vi "Oxford-IPS120-Main.vi"() -> ()   [LabVIEW 2013]
uses:
  <instrlib>/Mercury iXX/Public/Libraries/System/Read/Time (Read).vi
  <instrlib>/Mercury iXX/Public/Libraries/Temperature/Open/Open Temperature Device.vi
  <instrlib>/Mercury iXX/Public/Libraries/Magnet/Open/Open Magnet Device.vi
  <instrlib>/Mercury iXX/Public/Libraries/Level Meter/Open/Open Level Meter Device.vi
  <instrlib>/Mercury iXX/Public/Libraries/Magnet/Signals/Read/Switch Heater Status (Read).vi
  <instrlib>/Mercury iXX/Public/Libraries/Magnet/Signals/Read/Current (Read).vi
  <instrlib>/Mercury iXX/Public/Libraries/Magnet/Signals/Read/Persistant Current (Read).vi
  <instrlib>/Mercury iXX/Public/Libraries/Magnet/Configuration/Set/PSU Action Status (Set).vi
  <instrlib>/Mercury iXX/Public/Libraries/Magnet/Controls/PSU Actions.ctl
  <instrlib>/Mercury iXX/Public/Libraries/Magnet/Controls/Switch Heater.ctl
  <instrlib>/Mercury iXX/Public/Libraries/Magnet/Signals/Set/Switch Heater No Check (Set).vi
  <instrlib>/Mercury iXX/Public/Libraries/Magnet/Signals/Set/Target Field Rate (Set).vi
  <instrlib>/Mercury iXX/Public/Libraries/Magnet/Signals/Set/Target Field (Set).vi
  <instrlib>/Mercury iXX/Private/Controls/Command Verbs.ctl
  <instrlib>/Mercury iXX/Public/Controls/ISOBus Address.ctl
  <userlib>/_OpenG.lib/error/error.llb/Filter Error Codes (Array)__ogtk.vi
  <instrlib>/Mercury iXX/Public/Controls/Unit String.ctl
  <instrlib>/Mercury iXX/Public/Libraries/System/Open/Open Device.vi
panel:
  in  "IPS120 Address":refnum<visa-resource-name>="GPIB1::25::INSTR"
  out "LPF ON":timestamp
  in  "Tab Control":T1(tab)
  in  "Set Needle Valve (%)":dbl format="%_2g"
  out "Sentinel":bool=TRUE
  in  "Remote Mode":bool
  out "Power Supply Field (T)":dbl=0.0001 format="%#.5f"
  out "Magnet Field (T)":dbl format="%.5f"
  out "Voltage (V)":dbl=-0.0003 format="%.5f"
  out "Current (A)":dbl=0.0006 format="%.5f"
  in  "Fast/Slow Fill":bool
  in  "OK":bool
  out "Magnet Field (T)":dbl(knob) caption="Voltage (V)" scale=-20.0..20.0
  out "Magnet Status 2":string
  out "Switch Time":string="11:11:48"
  in  "PS Heat":bool
  in  "Clamp":bool
  in  "To Set":bool
  in  "To Zero":bool
  in  "Hold":bool
  out "Magnet Status":string="Clamped"
  out "Target Field Rate (T/min)":dbl=1.0 format="%.5f"
  out "Target Field (T)":dbl format="%#.5f"
  in  "Target Rate (T/min)":dbl=0.1 format="%.5f"
  in  "Target Field (T)":dbl format="%#.5f"
  in  "Send to IPS":bool
  out "Voltage (V)":dbl(knob)=-0.0003 scale=-10.0..10.0
  out "Current (A)":dbl(knob)=0.0006 scale=-180.0..180.0
  out "Error List":T2(array[cluster])
  in  "Lambda":bool
  out "LPF on (s)":i32=5373
  # "Voltage (V)"
  # "Magnet (T)"
  # "Current (A)"
  # "Slow Rates\nCurrent Range (A)     Field Range (T)    Rate (T/min)\n0       -- 100        0    -- 11.5       0.91\n100     -- 150        11.5 -- 17.2       0.23\n150     -- 155.467    17.2 -- 18         0.11\n155.567 -- 172.471    18   -- 20         0.11\n\nFast Rates\nCurrent Range (A)     Field Range (T)    Rate (T/min)\n0       -- 155.467    0    -- 18         1.0\n155.567 -- 172.471    18   -- 20         0.25"
  # "This Control Doesn't Work"
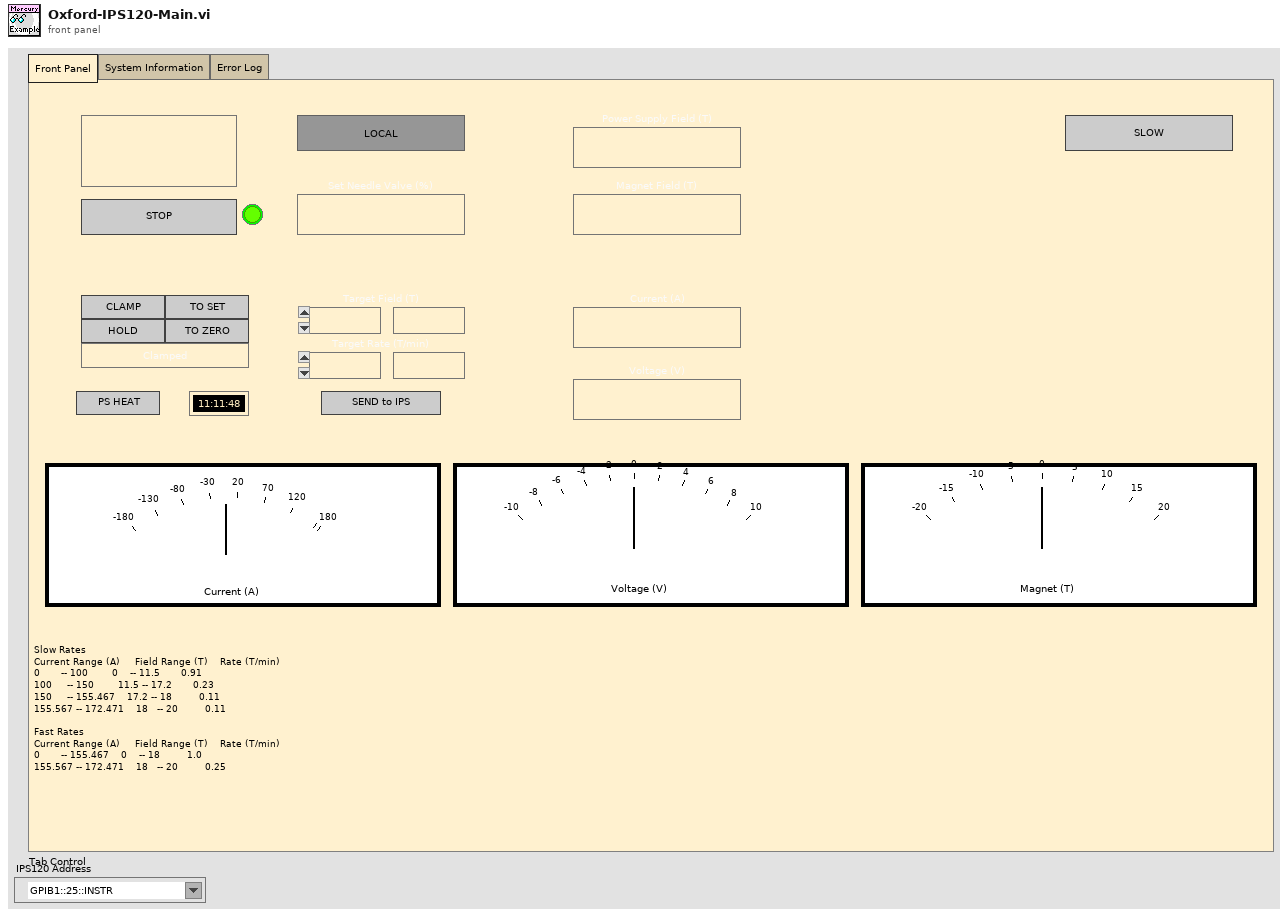
[diagram p1: front panel]
types:
  T1 = enum32{"Front Panel", "System Information", "Error Log"}
  T2 = cluster{"time":timestamp, "code":i32, "source":string}[]
  T3 = cluster{"Hold":bool, "Clamp":bool, "To Set":bool, "To Zero":bool, "Send to IPS":bool, "PS Heat":bool, "Lambda":bool}
  T4 = typedef "Mercury iXX.lvlib/Magnet.lvlib/PSU Actions.ctl" = string
  T5 = typedef "Mercury iXX.lvlib/Magnet.lvlib/Switch Heater.ctl" = string
  T6 = typedef "Mercury iXX.lvlib/Command Verbs.ctl" = string
  T7 = typedef "Mercury iXX.lvlib/ISOBus Address.ctl" = i32
  T8 = typedef "Mercury iXX.lvlib/Unit String.ctl" = string
  T9 = enum32{"invalid app kind", "Development System", "Run Time System", "Student Edition", "Embedded LabVIEW", "Evaluation", "Custom"}
  T10 = cluster{"time":timestamp, "code":i32, "source":string}
  T11 = enum32{"Invalid", "Standard", "Closed", "Hidden", "Minimized", "Maximized"}
  T12 = cluster{"Core":cluster{"Current VI Reference":refnum<vi>, "Close Panel on Exit?":bool}, "IPS120 Address":refnum<visa-resource-name>, "sentinel":bool, "Error Log":cluster{"time":timestamp, "code":i32, "source":string}[]}
  T13 = typedef "Mercury iXX.lvlib/Mercury Reference.ctl" = cluster{"Comms":refnum<visa-resource-name>, "Device ID":string[], "Comms Layer":T14, "Command":string, "Query reference":T15}
  T14 = typedef "Mercury iXX.lvlib/Comms Transport Layer.ctl" = enum16{"Ethernet TCP/IP", "USB", "ISOBus - RS-232", "GPIB"}
  T15 = typedef "Mercury iXX.lvlib/Query Dynamic Reference.ctl" = refnum<vi>
  T16 = typedef "Mercury iXX.lvlib/Response String.ctl" = string
  T17 = cluster{"Target Field (T)":dbl, "Target Field Rate (T/min)":dbl}
  T18 = typedef "Filtered Error Details - Cluster__ogtk.ctl" = cluster{"code":i32, "source":string}
  T19 = cluster{"Current VI Reference":refnum<vi>, "Close Panel on Exit?":bool}
  T20 = cluster{"Magnet Field":dbl, "PS Field":dbl, "Target Field":dbl, "Target Field Rate":dbl, "Voltage":dbl, "Current":dbl, "Switch":bool}
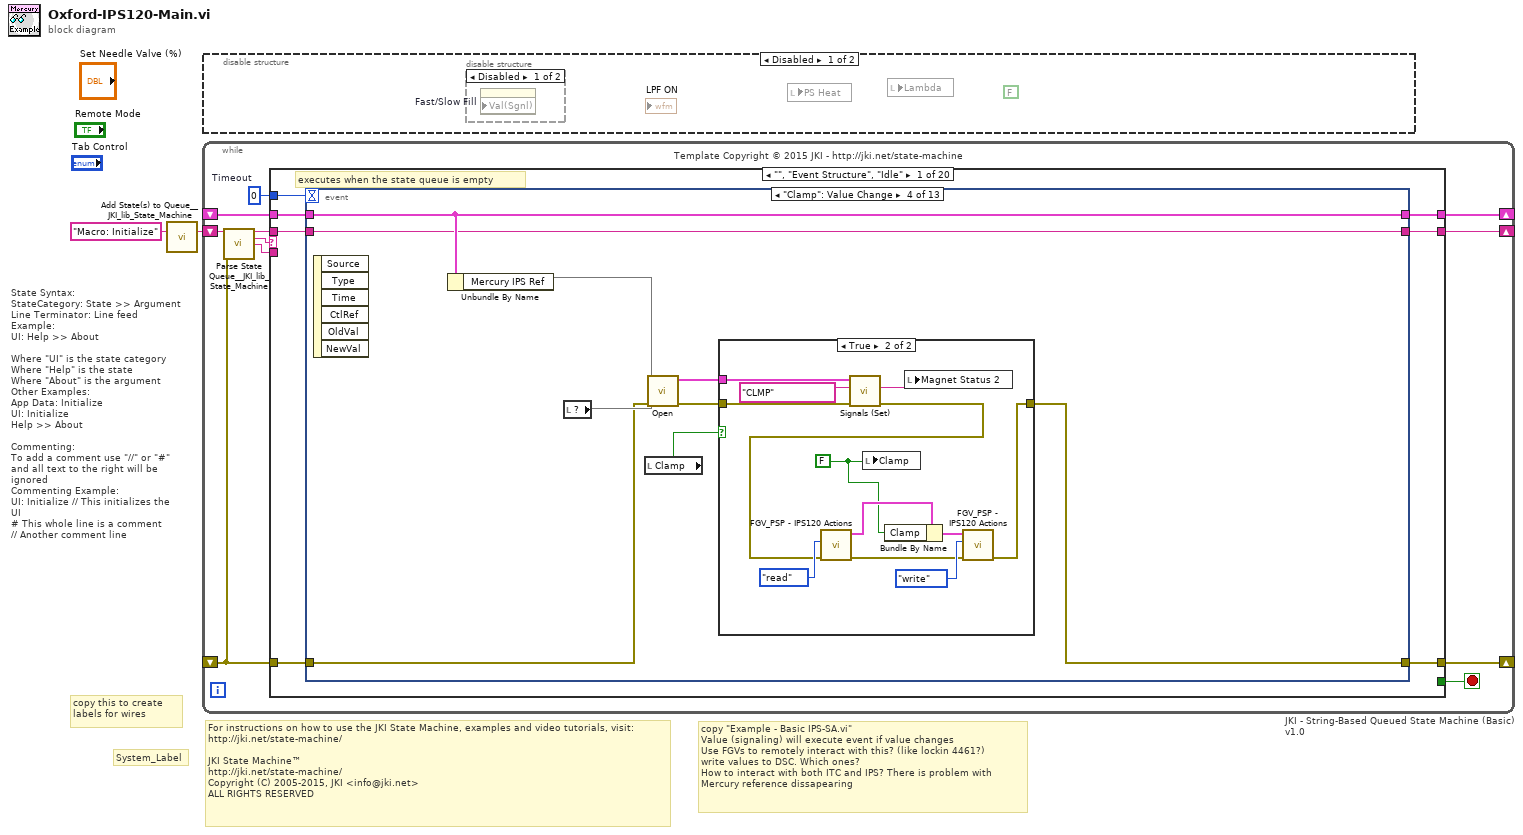
[diagram p0: block diagram]
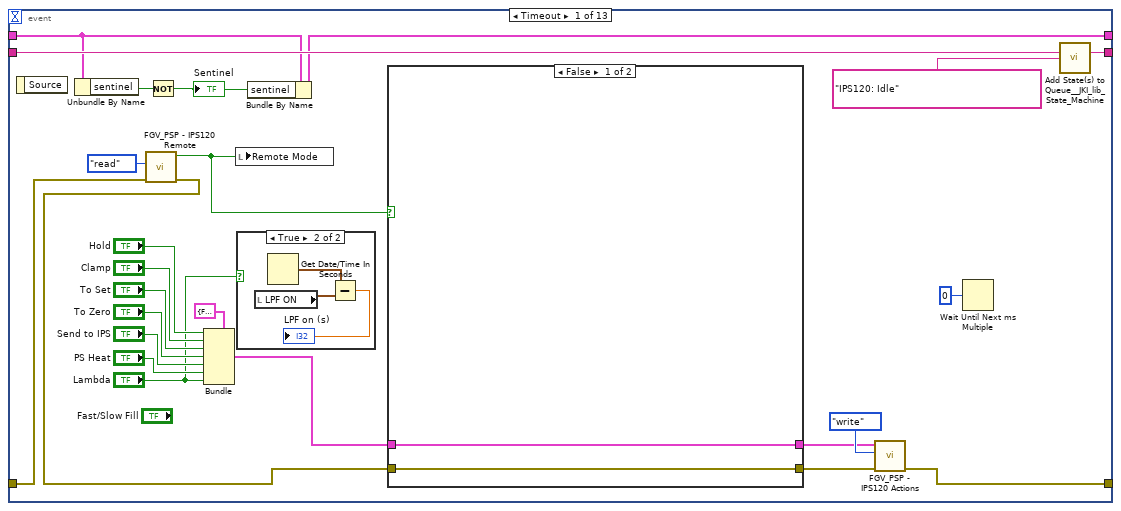
[diagram p4: hidden frame]
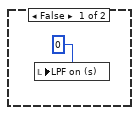
[diagram p5: hidden frame]
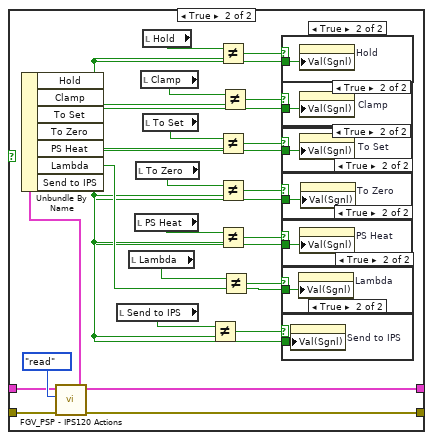
[diagram p6: hidden frame]
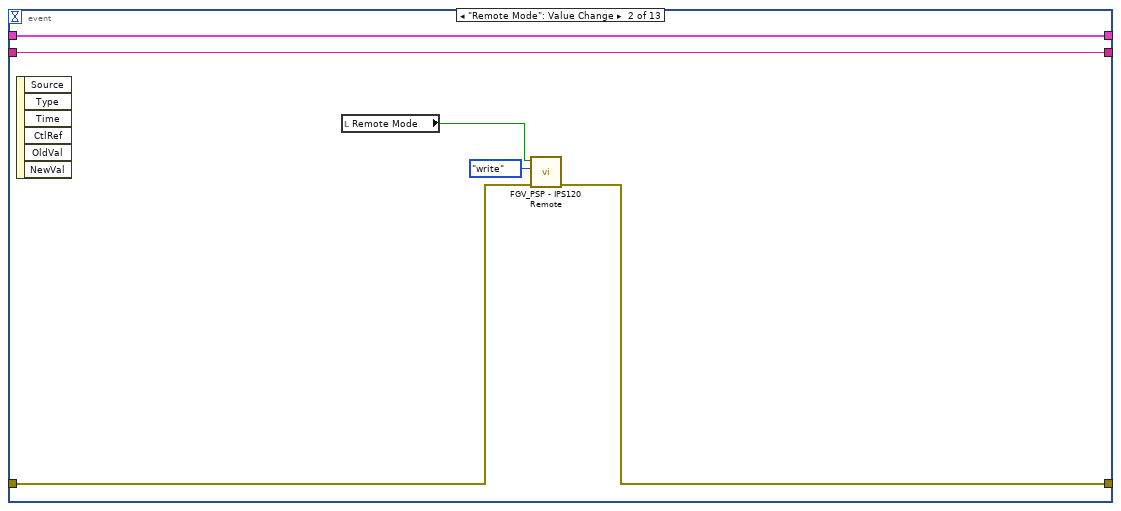
[diagram p14: hidden frame]
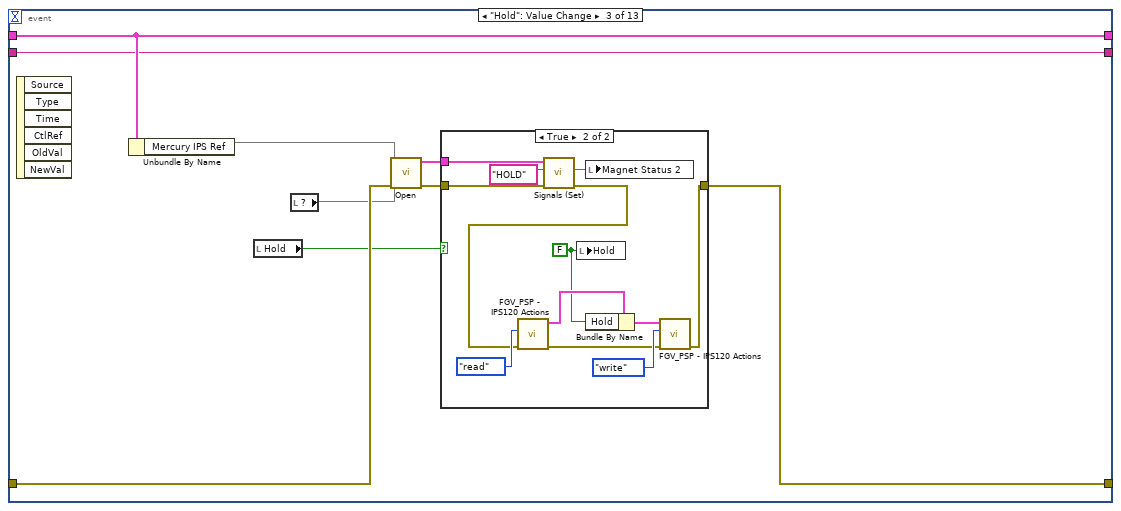
[diagram p15: hidden frame]
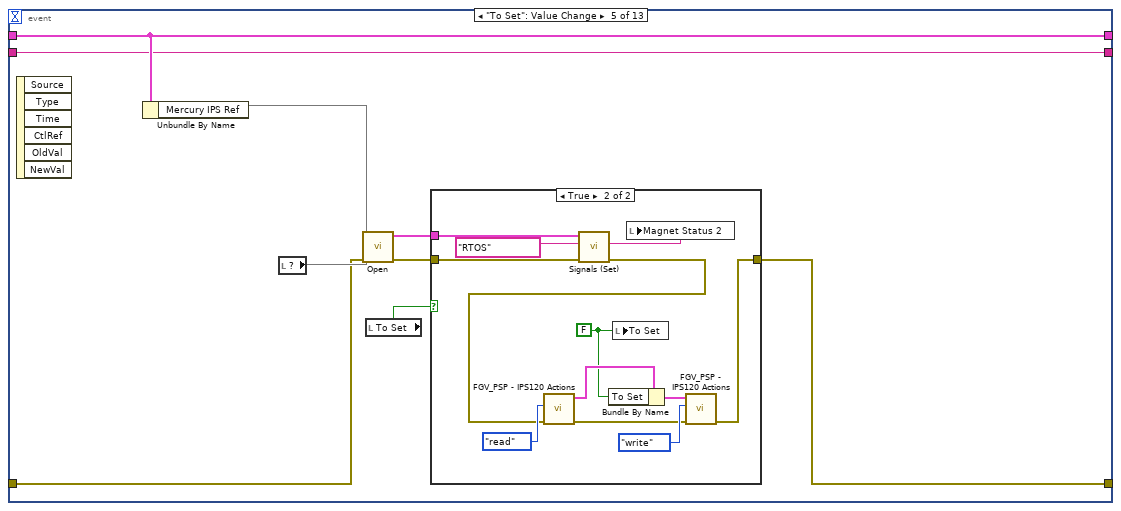
[diagram p18: hidden frame]
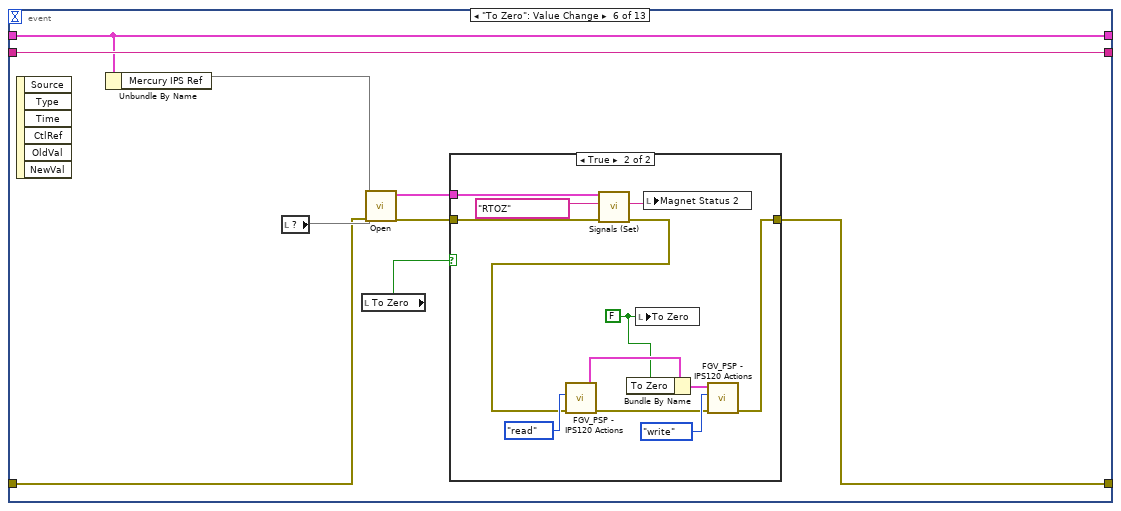
[diagram p20: hidden frame]
diagram:
  # "copy \"Example - Basic IPS-SA.vi\"\nValue (signaling) will execute event if value changes\nUse FGVs to remotely interact with this? (like lockin 4461?)\nwrite values to DSC. Which ones?\nHow to interact with both ITC and IPS? There is problem with \nMercury reference dissapearing"
  # "For instructions on how to use the JKI State Machine, examples and video tutorials, visit:\nhttp://jki.net/state-machine/\n\nJKI State Machine™\nhttp://jki.net/state-machine/\nCopyright (C) 2005-2015, JKI <info@jki.net>\nALL RIGHTS RESERVED"
  # "State Syntax:\nStateCategory: State >> Argument\nLine Terminator: Line feed\nExample:\nUI: Help >> About\n\nWhere \"UI\" is the state category\nWhere \"Help\" is the state\nWhere \"About\" is the argument\nOther Examples:\nApp Data: Initialize\nUI: Initialize\nHelp >> About\n\nCommenting:\nTo add a comment use \"//\" or \"#\" and all text to the right will be ignored\nCommenting Example:\nUI: Initialize // This initializes the UI\n# This whole line is a comment\n// Another comment line"
  # "copy this to create labels for wires"
  # "System_Label"
  n1 = call <vilib>:"Add State(s) to Queue__JKI_lib_State_Machine.vi"("State(s) in (\"\")"="Macro: Initialize") -> ("States Out"=w2:string)  [unwired: 14 in]
  n2 = while "JKI - String-Based Queued State Machine (Basic) v1.0" {
    shift-right: [w6] -> _
    shift-left: _ -> [w5]
    shift-right: [w9] -> _
    shift-left: _ -> [w3]
    shift-right: [w8] -> _
    shift-left: w2 -> [w10]
    stop <- w7 stop-if-true
    w4 = 0  # Timeout
    # "Template Copyright © 2015 JKI - http://jki.net/state-machine"
    n3 = call <vilib>:"Parse State Queue__JKI_lib_State_Machine.vi"("State Queue"=w10, "Error In (no error)"=w3) -> ("Remaining States"=w12:string, "Current State"=w13:string, "Arguments"=w11:string)  [unwired: 11 in]
    n4 = case shown="\"\", \"Event Structure\", \"Idle\"" w13 {
      selector: w13 -> [_ _ w361 _ _ _ _ _ _ _ _ _ _ _ _ _ _ _ _ _]
      tunnel: w12 -> [w20 w360 w365 w383 w400 w405 w409 w417 w423 w427 w439 w446 w457 w483 w488 w503 w507 w516 w551 w555]
      tunnel: w11 -> [_ _ _ _ _ _ _ _ _ _ _ w441 w451 _ _ _ _ _ _ _]
      tunnel: w5 -> [w16 w357 w363 w374 w386 w403 w406 _ w418 w424 w437 w444 w453 w480 w486 w501 w504 w514 w550 w554]
      tunnel: [w14 w358 w367 w380 errorcluster {"status"=FALSE, "code"=0, "source"=""} ("error out") w402 w407 w412 w419 w425 w433 w442 w454 w481 w485 w489 w505 w510 w546 w553] -> w9
      tunnel: [w19 w359 w364 w382 w399 w404 w408 w416 w422 w426 w438 w445 w456 w482 w487 w502 w506 w515 w552 w556] -> w8
      tunnel: [_ _ _ _ _ TRUE _ _ _ _ _ _ _ _ _ _ _ _ _ _] -> w7
      tunnel: [w18 w357 w363 w381 w385 w403 w406 w415 w418 w424 w437 w444 w453 w480 w486 w501 w504 w513 w550 w554] -> w6
      tunnel: w4 -> [w17 _ _ _ _ _ _ _ _ _ _ _ _ _ _ _ _ _ _ _]
      tunnel: w3 -> [w15 w358 w366 w380 w395 w402 w407 w412 w420 w425 w429 w443 w455 w481 w485 w491 w505 w511 w523 w553]
      frame "", "Event Structure", "Idle" {
        # "executes when the state queue is empty"
        n5 = event shown="[3] \"Clamp\": Value Change" {
          selector: _ -> [_ _ _ _ _ _ _ _ _ _ _ _ _]
          dyn-events: _ -> [_ _ _ _ _ _ _ _ _ _ _ _ _]
          timeout: w17 -> [_ _ _ _ _ _ _ _ _ _ _ _ _]
          tunnel: w20 -> [w45 w87 w98 w120 w141 w164 w190 w254 w285 w326 w329 w350 w356]
          tunnel: [w44 w87 w98 w120 w141 w164 w190 w254 w285 w326 w329 w349 w355] -> w19
          tunnel: [w39 w86 w99 w121 w142 w163 w191 w250 w284 w318 w344 w347 w353] -> w18
          tunnel: w16 -> [w40 w86 w99 w121 w142 w163 w191 w250 w284 w318 w344 w347 w353]
          tunnel: w15 -> [w23 w89 w95 w116 w136 w158 w184 w253 w282 w323 w331 w348 w354]
          tunnel: [w33 w88 w97 w113 w143 w165 w189 w251 w281 w306 w332 w348 w354] -> w14
          event Timeout {
            n6 = event-data() -> ()  [unwired: 1 in, 1 out]
            n7 = Unbundle By Name(w40) -> ("sentinel"=w42:bool)
            n8 = call "FGV_PSP - IPS120 Remote.vi"("error in"=w23, "Function"=enum16{"write", "read"}."read") -> ("error out"=w22:errorcluster, "Mercury Remote"=w21:bool)  [unwired: 4 in]
            n9 = Not(x=w42) -> (.not. x?=w41:bool)
            "Sentinel" <- w41
            n10 = Bundle(cluster=T3 {"Hold"=FALSE, "Clamp"=FALSE, "To Set"=FALSE, "To Zero"=FALSE, "Send to IPS"=FALSE, "PS Heat"=FALSE, "Lambda"=FALSE}, "Hold"="Hold", "Clamp"="Clamp", "To Set"="To Set", "To Zero"="To Zero", "Send to IPS"="Send to IPS", "PS Heat"="PS Heat", "Lambda"="Lambda") -> (w31:T3)
            n11 = local write "Remote Mode"(w21) -> ()
            n12 = case shown="True" "Lambda" {
              frame False {
                n13 = local write "LPF on (s)"(0 ("LPF on (s)")) -> ()
              }
              frame True {
                n14 = local read "LPF ON"() -> (w49:timestamp)
                n15 = Get Date/Time In Seconds() -> (seconds since 1Jan1904=w48:timestamp)
                n16 = Subtract(x=w48, y=w49) -> (x-y=→"LPF on (s)":dbl)
              }
            }
            n17 = Bundle By Name(cluster=w40, "sentinel"=w41) -> (w39:T12)
            n18 = case shown="False" w21 {
              tunnel: [w50 w76] -> w32
              tunnel: w22 -> [w50 w75]
              tunnel: w31 -> [w51 w74]
              tunnel: [w51 w66] -> w30
              frame False {
              }
              frame True {
                n19 = call "FGV_PSP - IPS120 Actions.vi"("error in"=w75, "Function"=enum16{"write", "read"}."read", "mercury actions"=w74) -> ("error out"=w76:errorcluster, "mercury actions 2"=w66:T3)  [unwired: 3 in]
                n20 = Unbundle By Name(w66) -> ("Hold"=w58:bool, "Clamp"=w60:bool, "To Set"=w61:bool, "To Zero"=w62:bool, "PS Heat"=w63:bool, "Lambda"=w64:bool, "Send to IPS"=w65:bool)
                n21 = local read "Send to IPS"() -> (w59:bool)
                n22 = local read "Lambda"() -> (w57:bool)
                n23 = local read "PS Heat"() -> (w56:bool)
                n24 = local read "To Zero"() -> (w55:bool)
                n25 = local read "Clamp"() -> (w53:bool)
                n26 = local read "Hold"() -> (w52:bool)
                n27 = local read "To Set"() -> (w54:bool)
                n28 = Not Equal?(x=w59, y=w65) -> (x != y?=w67:bool)
                n29 = Not Equal?(x=w52, y=w58) -> (x != y?=w73:bool)
                n30 = Not Equal?(x=w54, y=w61) -> (x != y?=w71:bool)
                n31 = Not Equal?(x=w55, y=w62) -> (x != y?=w70:bool)
                n32 = Not Equal?(x=w56, y=w63) -> (x != y?=w69:bool)
                n33 = Not Equal?(x=w53, y=w60) -> (x != y?=w72:bool)
                n34 = Not Equal?(x=w57, y=w64) -> (x != y?=w68:bool)
                n35 = case shown="True" w73 {
                  tunnel: w58 -> [_ w84]
                  frame False {
                  }
                  frame True {
                    n36 = property on="Hold" class="Bool (strict)"("Val(Sgnl)"=w84) -> ()  [unwired: 2 in, 2 out]
                  }
                }
                n37 = case shown="True" w72 {
                  tunnel: w60 -> [_ w83]
                  frame False {
                  }
                  frame True {
                    n38 = property on="Clamp" class="Bool (strict)"("Val(Sgnl)"=w83) -> ()  [unwired: 2 in, 2 out]
                  }
                }
                n39 = case shown="True" w71 {
                  tunnel: w61 -> [_ w82]
                  frame False {
                  }
                  frame True {
                    n40 = property on="To Set" class="Bool (strict)"("Val(Sgnl)"=w82) -> ()  [unwired: 2 in, 2 out]
                  }
                }
                n41 = case shown="True" w70 {
                  tunnel: w62 -> [_ w81]
                  frame False {
                  }
                  frame True {
                    n42 = property on="To Zero" class="Bool (strict)"("Val(Sgnl)"=w81) -> ()  [unwired: 2 in, 2 out]
                  }
                }
                n43 = case shown="True" w69 {
                  tunnel: w63 -> [_ w80]
                  frame False {
                  }
                  frame True {
                    n44 = property on="PS Heat" class="Bool (strict)"("Val(Sgnl)"=w80) -> ()  [unwired: 2 in, 2 out]
                  }
                }
                n45 = case shown="True" w68 {
                  tunnel: w64 -> [_ w79]
                  frame False {
                  }
                  frame True {
                    n46 = property on="Lambda" class="Bool (strict)"("Val(Sgnl)"=w79) -> ()  [unwired: 2 in, 2 out]
                  }
                }
                n47 = case shown="True" w67 {
                  tunnel: w65 -> [_ w78]
                  frame False {
                  }
                  frame True {
                    n48 = property on="Send to IPS" class="Bool (strict)"("Val(Sgnl)"=w78) -> ()  [unwired: 2 in, 2 out]
                  }
                }
              }
            }
            n49 = call "FGV_PSP - IPS120 Actions.vi"("error in"=w32, "Function"=enum16{"write", "read"}."write", "mercury actions"=w30) -> ("error out"=w33:errorcluster)  [unwired: 3 in, 1 out]
            n50 = Wait Until Next ms Multiple(millisecond multiple=u32 0) -> ()  [unwired: 1 out]
            n51 = call <vilib>:"Add State(s) to Queue__JKI_lib_State_Machine.vi"("State(s) in (\"\")"=w45, "State(s) at Back (\"\")"="IPS120: Idle" ("State(s) at Back (\"\")")) -> ("States Out"=w44:string)  [unwired: 13 in]
          }
          event "Remote Mode": Value Change {
            n52 = event-data() -> ()  [unwired: 1 in, 6 out]
            n53 = local read "Remote Mode"() -> (w85:bool)
            n54 = call "FGV_PSP - IPS120 Remote.vi"("error in"=w89, "Function"=enum16{"write", "read"}."write", "Mercury Remote"=w85) -> ("error out"=w88:errorcluster)  [unwired: 3 in, 1 out]
          }
          event "Hold": Value Change {
            n55 = event-data() -> ()  [unwired: 1 in, 6 out]
            n56 = Unbundle By Name(w99) -> ("Mercury IPS Ref"=w93)
            n57 = local read "Hold"() -> (w91:bool)
            n58 = local read item#-1() -> (w94)
            n59 = call-poly <instrlib>:"Open.vi"("error in (no error)"=w95, "Device Identifier"=w94, "Mercury Reference In"=w93) -> ("error out"=w96:errorcluster, "Mercury Reference Out"=w92:T13)  [unwired: 7 out]
            n60 = case shown="True" w91 {
              tunnel: [w100 w102] -> w97
              tunnel: w96 -> [w100 w111]
              tunnel: w92 -> [_ w110]
              frame False {
              }
              frame True {
                w107 = FALSE ("Hold")
                n61 = call-poly <instrlib>:"Signals (Set).vi"("error in"=w111, "PSU Act Stat"=T4 "HOLD", "Mercury Reference In"=w110) -> ("error out"=w101:errorcluster, "Response"=w109:T16)  [unwired: 1 in, 6 out]
                n62 = call "FGV_PSP - IPS120 Actions.vi"("error in"=w101, "Function"=enum16{"write", "read"}."read") -> ("error out"=w104:errorcluster, "mercury actions 2"=w108:T3)  [unwired: 4 in]
                n63 = local write "Hold"(w107) -> ()
                n64 = local write "Magnet Status 2"(w109) -> ()
                n65 = Bundle By Name(cluster=w108, "Hold"=w107) -> (w106:T3)
                n66 = call "FGV_PSP - IPS120 Actions.vi"("error in"=w104, "Function"=enum16{"write", "read"}."write", "mercury actions"=w106) -> ("error out"=w102:errorcluster)  [unwired: 3 in, 1 out]
              }
            }
          }
          event "Clamp": Value Change {
            n67 = event-data() -> ()  [unwired: 1 in, 6 out]
            n68 = Unbundle By Name(w121) -> ("Mercury IPS Ref"=w115)
            n69 = local read item#-1() -> (w119)
            n70 = local read "Clamp"() -> (w114:bool)
            n71 = call-poly <instrlib>:"Open.vi"("error in (no error)"=w116, "Device Identifier"=w119, "Mercury Reference In"=w115) -> ("error out"=w118:errorcluster, "Mercury Reference Out"=w117:T13)  [unwired: 7 out]
            n72 = case shown="True" w114 {
              tunnel: w118 -> [w122 w132]
              tunnel: w117 -> [_ w131]
              tunnel: [w122 w124] -> w113
              frame False {
              }
              frame True {
                w123 = FALSE
                n73 = call-poly <instrlib>:"Signals (Set).vi"("error in"=w132, "PSU Act Stat"=T4 "CLMP", "Mercury Reference In"=w131) -> ("error out"=w125:errorcluster, "Response"=w133:T16)  [unwired: 1 in, 6 out]
                n74 = call "FGV_PSP - IPS120 Actions.vi"("error in"=w125, "Function"=enum16{"write", "read"}."read") -> ("error out"=w127:errorcluster, "mercury actions 2"=w130:T3)  [unwired: 4 in]
                n75 = local write "Clamp"(w123) -> ()
                n76 = Bundle By Name(cluster=w130, "Clamp"=w123) -> (w129:T3)
                n77 = local write "Magnet Status 2"(w133) -> ()
                n78 = call "FGV_PSP - IPS120 Actions.vi"("error in"=w127, "Function"=enum16{"write", "read"}."write", "mercury actions"=w129) -> ("error out"=w124:errorcluster)  [unwired: 3 in, 1 out]
              }
            }
          }
          event "To Set": Value Change {
            n79 = event-data() -> ()  [unwired: 1 in, 6 out]
            n80 = Unbundle By Name(w142) -> ("Mercury IPS Ref"=w138)
            n81 = local read item#-1() -> (w137)
            n82 = call-poly <instrlib>:"Open.vi"("error in (no error)"=w136, "Device Identifier"=w137, "Mercury Reference In"=w138) -> ("error out"=w139:errorcluster, "Mercury Reference Out"=w140:T13)  [unwired: 7 out]
            n83 = local read "To Set"() -> (w135:bool)
            n84 = case shown="True" w135 {
              tunnel: [w144 w146] -> w143
              tunnel: w140 -> [_ w154]
              tunnel: w139 -> [w144 w153]
              frame False {
              }
              frame True {
                w145 = FALSE
                n85 = call-poly <instrlib>:"Signals (Set).vi"("error in"=w153, "PSU Act Stat"=T4 "RTOS", "Mercury Reference In"=w154) -> ("error out"=w147:errorcluster, "Response"=w155:T16)  [unwired: 1 in, 6 out]
                n86 = call "FGV_PSP - IPS120 Actions.vi"("error in"=w147, "Function"=enum16{"write", "read"}."read") -> ("error out"=w149:errorcluster, "mercury actions 2"=w152:T3)  [unwired: 4 in]
                n87 = Bundle By Name(cluster=w152, "To Set"=w145) -> (w151:T3)
                n88 = local write "To Set"(w145) -> ()
                n89 = local write "Magnet Status 2"(w155) -> ()
                n90 = call "FGV_PSP - IPS120 Actions.vi"("error in"=w149, "Function"=enum16{"write", "read"}."write", "mercury actions"=w151) -> ("error out"=w146:errorcluster)  [unwired: 3 in, 1 out]
              }
            }
          }
          event "To Zero": Value Change {
            n91 = event-data() -> ()  [unwired: 1 in, 6 out]
            n92 = Unbundle By Name(w163) -> ("Mercury IPS Ref"=w160)
            n93 = local read item#-1() -> (w159)
            n94 = local read "To Zero"() -> (w157:bool)
            n95 = call-poly <instrlib>:"Open.vi"("error in (no error)"=w158, "Device Identifier"=w159, "Mercury Reference In"=w160) -> ("error out"=w161:errorcluster, "Mercury Reference Out"=w162:T13)  [unwired: 7 out]
            n96 = case shown="True" w157 {
              tunnel: [w166 w169] -> w165
              tunnel: w162 -> [_ w176]
              tunnel: w161 -> [w166 w175]
              frame False {
              }
              frame True {
                w167 = FALSE
                n97 = call-poly <instrlib>:"Signals (Set).vi"("error in"=w175, "PSU Act Stat"=T4 "RTOZ", "Mercury Reference In"=w176) -> ("error out"=w170:errorcluster, "Response"=w177:T16)  [unwired: 1 in, 6 out]
                n98 = call "FGV_PSP - IPS120 Actions.vi"("error in"=w170, "Function"=enum16{"write", "read"}."read") -> ("error out"=w172:errorcluster, "mercury actions 2"=w168:T3)  [unwired: 4 in]
                n99 = Bundle By Name(cluster=w168, "To Zero"=w167) -> (w174:T3)
                n100 = local write "To Zero"(w167) -> ()
                n101 = local write "Magnet Status 2"(w177) -> ()
                n102 = call "FGV_PSP - IPS120 Actions.vi"("error in"=w172, "Function"=enum16{"write", "read"}."write", "mercury actions"=w174) -> ("error out"=w169:errorcluster)  [unwired: 3 in, 1 out]
              }
            }
          }
          event "PS Heat": Value Change {
            n103 = event-data() -> ()  [unwired: 1 in, 6 out]
            n104 = local read item#-1() -> (w185)
            n105 = Unbundle By Name(w191) -> ("Mercury IPS Ref"=w187)
            n106 = call-poly <instrlib>:"Open.vi"("error in (no error)"=w184, "Device Identifier"=w185, "Mercury Reference In"=w187) -> ("error out"=w181:errorcluster, "Mercury Reference Out"=w182:T13)  [unwired: 7 out]
            n107 = call-poly <instrlib>:"Signals (Read).vi"("error in"=w181, "Mercury Reference In"=w182) -> ("error out"=w193:errorcluster, "Current"=w188:dbl, "Mercury Reference Out"=w192:T13)  [unwired: 1 in, 6 out]
            n108 = local read "PS Heat"() -> (w180:bool)
            n109 = call-poly <instrlib>:"Signals (Read).vi"("error in"=w193, "Mercury Reference In"=w192) -> ("error out"=w194:errorcluster, "Persistant Current"=w183:dbl, "Mercury Reference Out"=w195:T13)  [unwired: 1 in, 6 out]
            n110 = Subtract(x=w183, y=w188) -> (x-y=w196:dbl)
            n111 = Absolute Value(x=w196) -> (abs(x)=w197:dbl)
            n112 = Less?(x=w197, y=0.1) -> (x < y?=w199:bool)
            n113 = case shown="False" w199 {
              selector: w199 -> [_ w202]
              tunnel: [w201 w202] -> w179
              frame False {
                n114 = Two Button Dialog(message="The magnet current is more\nthan 0.1A different to the\nPSU output current.  It is not\nadvisable to switch on the\nswitch heater unless these\ncurrents are equal!") -> (T button?=w201:bool)  [unwired: 2 out]
              }
              frame True {
              }
            }
            n115 = And(x=w180, y=w179) -> (x .and. y?=w186:bool)
            n116 = case shown="True" w186 {
              tunnel: w195 -> [_ w213]
              tunnel: w194 -> [w203 w212]
              tunnel: [w203 w204] -> w189
              frame False {
              }
              frame True {
                w206 = FALSE
                n117 = flat-sequence {
                  tunnel: [w224] -> w221
                  tunnel: [w223] -> w220
                  tunnel: [w222] -> w219
                  tunnel: w213 -> [w226]
                  tunnel: w212 -> [w225]
                  tunnel: w221 -> [w229]
                  tunnel: w220 -> [w228]
                  tunnel: [w229] -> w218
                  tunnel: [w228] -> w217
                  tunnel: [w227] -> w216
                  tunnel: w219 -> [w227]
                  tunnel: w218 -> [w240]
                  tunnel: w217 -> [w241]
                  tunnel: w216 -> [w238]
                  tunnel: [w235] -> w215
                  tunnel: [w236] -> w214
                  tunnel: w215 -> [w245]
                  tunnel: w214 -> [w244]
                  tunnel: [w243] -> w205
                  frame #0 {
                    n118 = call-poly <instrlib>:"Signals (Read).vi"("error in"=w225, "Mercury Reference In"=w226) -> ("error out"=w224:errorcluster, "Switch Heater Status"=w222:string, "Mercury Reference Out"=w223:T13)  [unwired: 1 in, 6 out]
                  }
                  frame #1 {
                    n119 = Wait Until Next ms Multiple(millisecond multiple=u32 100) -> ()  [unwired: 1 out]
                  }
                  frame #2 {
                    n120 = Equal?(x=w238, y="ON") -> (x = y?=w237:bool)
                    n121 = Select(t=T5 "OFF" ("Set Switch Heater"), s=w237, f=T5 "ON" ("Set Switch Heater")) -> (s? t:f=w232:T5)
                    n122 = call-poly <instrlib>:"Signals (Set).vi"("error in"=w240, "Set Switch Heater"=w232, "Mercury Reference In"=w241) -> ("error out"=w236:errorcluster, "Response"=w231:T16, "Mercury Reference Out"=w235:T13)  [unwired: 1 in, 5 out]
                    n123 = local write "Magnet Status 2"(w231) -> ()
                  }
                  frame #3 {
                    n124 = call-poly <instrlib>:"Configuration (Read).vi"("error in"=w244, "Mercury Reference In"=w245) -> ("error out"=w243:errorcluster, "Time"=→"Switch Time":string)  [unwired: 1 in, 7 out]
                  }
                }
                n125 = call "FGV_PSP - IPS120 Actions.vi"("error in"=w205, "Function"=enum16{"write", "read"}."read") -> ("error out"=w209:errorcluster, "mercury actions 2"=w207:T3)  [unwired: 4 in]
                n126 = local write "PS Heat"(w206) -> ()
                n127 = Bundle By Name(cluster=w207, "PS Heat"=w206) -> (w211:T3)
                n128 = call "FGV_PSP - IPS120 Actions.vi"("error in"=w209, "Function"=enum16{"write", "read"}."write", "mercury actions"=w211) -> ("error out"=w204:errorcluster)  [unwired: 3 in, 1 out]
              }
            }
          }
          event "Send to IPS": Value Change {
            n129 = event-data() -> ()  [unwired: 1 in, 6 out]
            n130 = Unbundle By Name(w250) -> ("Mercury IPS Ref"=w248)
            n131 = local read item#-1() -> (w249)
            n132 = local read "Send to IPS"() -> (w246:bool)
            n133 = call-poly <instrlib>:"Open.vi"("error in (no error)"=w253, "Device Identifier"=w249, "Mercury Reference In"=w248) -> ("error out"=w252:errorcluster, "Mercury Reference Out"=w247:T13)  [unwired: 7 out]
            n134 = case shown="True" w246 {
              tunnel: w252 -> [w255 w274]
              tunnel: [w255 w258] -> w251
              tunnel: w247 -> [_ w272]
              frame False {
              }
              frame True {
                w257 = FALSE
                n135 = local read "Remote Mode"() -> (w270:bool)
                n136 = case shown="True" w270 {
                  tunnel: "Target Field (T)" -> [w276 _]
                  tunnel: "Target Rate (T/min)" -> [w275 _]
                  tunnel: [w276 w278] -> w264
                  tunnel: [w275 w277] -> w265
                  frame False {
                  }
                  frame True {
                    n137 = call "FGV_PSP - IPS120 Targets.vi"("Function"=enum16{"write", "read"}."read") -> ("Mercury Targets"=w279:T17)  [unwired: 5 in, 1 out]
                    n138 = Unbundle(w279) -> ("Target Field (T)"=w278:dbl, "Target Field Rate (T/min)"=w277:dbl)
                  }
                }
                n139 = local write "Send to IPS"(w257) -> ()
                n140 = call-poly <instrlib>:"Signals (Set).vi"("error in"=w274, "Target Field Rate"=w265, "Mercury Reference In"=w272) -> ("error out"=w273:errorcluster, "Mercury Reference Out"=w271:T13)  [unwired: 2 in, 5 out]
                n141 = local write "Target Field (T)"(w264) -> ()
                n142 = local write "Target Rate (T/min)"(w265) -> ()
                n143 = Bundle("Target Field (T)"=w264, "Target Field Rate (T/min)"=w265) -> (w267:T17)  [unwired: 1 in]
                n144 = call-poly <instrlib>:"Signals (Set).vi"("error in"=w273, "Target Field"=w264, "Mercury Reference In"=w271) -> ("error out"=w256:errorcluster)  [unwired: 2 in, 6 out]
                n145 = call "FGV_PSP - IPS120 Actions.vi"("error in"=w256, "Function"=enum16{"write", "read"}."read") -> ("error out"=w261:errorcluster, "mercury actions 2"=w259:T3)  [unwired: 4 in]
                n146 = Bundle By Name(cluster=w259, "Send to IPS"=w257) -> (w263:T3)
                n147 = call "FGV_PSP - IPS120 Actions.vi"("error in"=w261, "Function"=enum16{"write", "read"}."write", "mercury actions"=w263) -> ("error out"=w258:errorcluster)  [unwired: 3 in, 1 out]
                n148 = call "FGV_PSP - IPS120 Targets.vi"("Function"=enum16{"write", "read"}."write", "Mercury Targets"=w267) -> ()  [unwired: 4 in, 2 out]
              }
            }
          }
          event "Lambda": Value Change {
            n149 = event-data() -> ()  [unwired: 1 in, 6 out]
            n150 = Unbundle By Name(w284) -> ("Mercury ITC Ref"=w283)
            n151 = disable-structure shown="Disabled" {
              disable-tunnel: w283 -> [w302 _]
              disable-tunnel: w282 -> [w299 _]
              disable-tunnel: [w287 _] -> w281
              frame Disabled {
                # "TEMP device"
                # "AUX\nPRES\nHTR\nTEMP"
                n152 = local read item#-1() -> (w303)
                n153 = Index Array(array=w303, index=3 ("Lambda device")) -> (element=w301)
                n154 = call-poly <instrlib>:"Open.vi"("error in (no error)"=w299, "Device Identifier"=w301, "Mercury Reference In"=w302) -> ("error out"=w291:errorcluster, "Mercury Reference Out"=w290:T13)  [unwired: 1 in, 6 out]
                n155 = local read "Lambda"() -> (w298:bool)
                n156 = call <instrlib>:"Build SCPI Command.vi"("error in"=w291, "Noun(s)"=":SIG:PERC:", "Verb"=T6 "SET:", "Mercury Reference In"=w290) -> ("error out"=w288:errorcluster, "SCPI Message(s)"=w292:string[], "Mercury Reference Out"=w294:T13)  [unwired: 5 in]
                n157 = Select(t="ON" ("Sweep Mode"), s=w298, f="OFF" ("Sweep Mode")) -> ()  [unwired: 1 out]
                n158 = case shown="True" w298 {
                  frame False {
                    n159 = local write "LPF ON"(timestamp(0 s since 1904-01-01) ("LPF ON")) -> ()
                  }
                  frame True {
                    n160 = Get Date/Time In Seconds() -> (seconds since 1Jan1904=w305:timestamp)
                    n161 = local write "LPF ON"(w305) -> ()
                  }
                }
                n162 = call <instrlib>:"Set (Str).vi"("ISOBUS address"=T7 -1, "error in"=w288, "SCPI Message(s)"=w292, "Mercury Reference In"=w294) -> ("error out"=w287:errorcluster, "Response"=w286:T16)  [unwired: 4 in, 2 out]
                n163 = local write "Magnet Status 2"(w286) -> ()
              }
              frame Enabled {
              }
            }
          }
          event "Fast/Slow Fill": Value Change {
            n164 = event-data() -> ()  [unwired: 1 in, 6 out]
            n165 = local read item#-1() -> (w320)
            n166 = Unbundle By Name(w318) -> ("Mercury IPS Ref"=w325)
            n167 = Index Array(array=w320, index=0) -> (element=w319)
            n168 = call-poly <instrlib>:"Open.vi"("error in (no error)"=w323, "Device Identifier"=w319, "Mercury Reference In"=w325) -> ("error out"=w316:errorcluster, "Mercury Reference Out"=w324:T13)  [unwired: 7 out]
            n169 = local read "Fast/Slow Fill"() -> (w311:bool)
            n170 = call <instrlib>:"Build SCPI Command.vi"("error in"=w316, "Noun(s)"=":HEL:PULS:SLOW:", "Verb"=T6 "SET:", "Mercury Reference In"=w324) -> ("error out"=w309:errorcluster, "SCPI Message(s)"=w314:string[], "Mercury Reference Out"=w308:T13)  [unwired: 5 in]
            n171 = Select(t="OFF" ("Temperature setpoint"), s=w311, f="ON" ("Temperature setpoint")) -> (s? t:f=w313:string)
            n172 = call <instrlib>:"Set (Str).vi"("ISOBUS address"=T7 -1, "error in"=w309, "Command Value (Str)"=w313, "SCPI Message(s)"=w314, "Mercury Reference In"=w308) -> ("error out"=w306:errorcluster, "Response"=w307:T16)  [unwired: 5 out]
            n173 = local write "Magnet Status 2"(w307) -> ()
          }
          event "Set Needle Valve (%)": Value Change {
            n174 = event-data() -> ("NewVal"=w333:dbl)  [unwired: 1 in, 5 out]
            n175 = Unbundle By Name(w344) -> ("Mercury ITC Ref"=w345)
            n176 = local read item#-1() -> (w342)
            n177 = Index Array(array=w342, index=3) -> (element=w341)
            n178 = call-poly <instrlib>:"Open.vi"("error in (no error)"=w331, "Device Identifier"=w341, "Mercury Reference In"=w345) -> ("error out"=w335:errorcluster, "Mercury Reference Out"=w334:T13)  [unwired: 7 out]
            n179 = call <instrlib>:"Build SCPI Command.vi"("error in"=w335, "Noun(s)"=":LOOP:FSET:", "Verb"=T6 "SET:", "Mercury Reference In"=w334) -> ("error out"=w336:errorcluster, "SCPI Message(s)"=w327:string[], "Mercury Reference Out"=w338:T13)  [unwired: 5 in]
            n180 = call <instrlib>:"Set (DBL).vi"("ISOBUS address"=T7 -1, "Unit"=T8 "", "error in"=w336, "Command Value (Dbl)"=w333, "SCPI Message(s)"=w327, "Mercury Reference In"=w338) -> ("error out"=w332:errorcluster, "Response"=w328:T16)  [unwired: 2 in, 2 out]
            n181 = local write "Magnet Status 2"(w328) -> ()
          }
          event "OK": Value Change {
            # "Exit Button Value Change (pressed) Event\n(this executes Macro: Exit to terminate the VI)"
            n182 = event-data() -> ()  [unwired: 1 in, 1 out]
            n183 = call <vilib>:"Add State(s) to Queue__JKI_lib_State_Machine.vi"("State(s) in Front (\"\")"="Macro: Exit", "State(s) in (\"\")"=w350) -> ("States Out"=w349:string)  [unwired: 13 in]
          }
          event Panel Close? {
            # "Discard the event because we'll close the front panel ourselves in Macro: Exit"
            # "Close Panel button (pressed) Event\n(this executes Macro: Exit to terminate the VI)"
            n184 = event-data() -> ()  [unwired: 1 in, 1 out]
            n185 = call <vilib>:"Add State(s) to Queue__JKI_lib_State_Machine.vi"("State(s) in Front (\"\")"="Macro: Exit", "State(s) in (\"\")"=w356) -> ("States Out"=w355:string)  [unwired: 13 in]
            n186 = event-data("Discard?"=TRUE) -> ()  [unwired: 1 in, 1 out]
          }
        }
      }
      frame "---------- Core ----------" {
        # "Do not put any code in this frame.\n(it is a separator no-op)"
        n187 = call <vilib>:"Add State(s) to Queue__JKI_lib_State_Machine.vi"("State(s) in (\"\")"=w360) -> ("States Out"=w359:string)  [unwired: 14 in]
      }
      frame Default {
        w370 = 42 items=["No error", "Argument error", "Memory is full", "Out of zone", "End of file", "File already open", "Generic file I/O error", "File not found", "File permission error", "Disk is full", "Duplicate path", "Too many files open", "System feature not enabled", "Resource file not found", "Cannot add resource", "Resource not found", "Image not found", "Image memory error", "Pen does not exist", "Config type invalid", "Config token not found", "Config parse error", "Config memory error", "Bad external code format", "Bad external code offset", "External code not present", "Null window", "Destroy window error", "Null menu", "Print aborted", "Bad print record", "Print driver error", "Windows error during printing", "Memory error during printing", "Print dialog error", "Generic print error", "Invalid device refnum", "Device not found", "Device parameter error", "Device unit error", "Cannot open device", "Device call aborted", "Generic error", "Cancelled by user", "Object ID too low", "Object ID too high", "Object not in heap", "Unknown heap", "Unknown object (invalid DefProc)", "Unknown object (DefProc not in table)", "Message out of range", "Invalid (null) method", "Unknown message", "Manager call not supported", "Bad address", "Network operation in progress", "Network operation timed out", "Connection is busy", "Network attribute not supported", "Network error", "Address in use", "System out of memory", "Connection aborted", "Connection refused", "Not connected", "Already connected", "Connection closed", "Initialization error (interapplication manager)", "Bad occurrence", "Wait on unbound occurrence handler", "Occurrence queue overflow", "Datalog type conflict", "Unused", "Unrecognized type (interapplication manager)", "Memory corrupt", "Failed to make temporary DLL", "Old CIN version", "Drag socket not found", "Failed to load drop-object", "Failed to register OLE object", "Failed to release OLE object", "Format specifier type mismatch", "Unknown format specifier", "Too few format specifiers", "Too many format specifiers", "Scan failed", "Newer CIN version", "Error converting to variant", "Runtime menu error", "Password tampered", "Variant attribute not found", "Incompatible variant data type", "Event data is not available", "Event Store is not present", "Occurrence is not found", "Event Queue is not created", "Event info is not available", "Refnum passed is NULL", "Error retrieving Class GUID", "Error retrieving CoClass GUID", "Error retrieving TypeLib GUID.", "Bad built application magic bytes.", "Specific driver is different from the specific driver associated with the Logical Name.", "There is no session opened to the class driver.", "Max Error", "MAX - Error with config objects", "MAX - Error loading configuration", "MAX - Group not supported"]
        # "Current State"
        # "Do not delete, rename, or modify this frame.\n(this is used to capture unhandled states and typos)"
        # "Handle mistyped state name (developer tool)"
        n188 = Format Into String(format string="Software Exception: Unhandled State \"%s\"." ("message"), error in=w366, w361) -> (resulting string=w369:string, error out=w368:errorcluster)  [unwired: 1 in]
        n189 = call <vilib>:"Error Cluster From Error Code.vi"("show call chain? (False)"=TRUE, "error in (no error)"=w368, "error message (\"\")"=w369, "error code (0)"=w370) -> ("error out"=w367:errorcluster)  [unwired: 5 in]
        n190 = call <vilib>:"Add State(s) to Queue__JKI_lib_State_Machine.vi"("State(s) in (\"\")"=w365) -> ("States Out"=w364:string)  [unwired: 14 in]
      }
      frame "Initialize Core Data" {
        # "Do not delete, rename, or modify this frame.\n(this is used to determine panel behavior on exit)"
        # "originally closed?"
        # "exe?"
        # "If panel starts closed or is an EXE, then close it when we exit"
        n191 = property class="VI"() -> ("Front Panel.Open"=w379:bool)  [unwired: 2 in, 2 out]
        n192 = property class="App"() -> ("App.Kind"=w378:T9)  [unwired: 2 in, 2 out]
        n193 = control-ref of="Current VI Reference"() -> (w372:refnum<vi>)
        n194 = Not(x=w379) -> (.not. x?=w376:bool)
        n195 = Equal?(x=w378, y=T9."Run Time System" ("Application:Kind")) -> (x = y?=w375:bool)
        n196 = Or(x=w376, y=w375) -> (x .or. y?=w373:bool)
        n197 = Bundle By Name(cluster=w374, "Core.Current VI Reference"=w372, "Core.Close Panel on Exit?"=w373) -> (w381:T12)
        n198 = call <vilib>:"Add State(s) to Queue__JKI_lib_State_Machine.vi"("State(s) in (\"\")"=w383) -> ("States Out"=w382:string)  [unwired: 14 in]
      }
      frame "Error Handler" {
        w394 = i32[] [-1950679035, -1950678943]  # Error Codes to Filter
        # "Unhandled Error -- Display it"
        # "Handle any errors here.\nYou can also output any states to clean-up after errors occur"
        # "Clear error"
        n199 = call-poly <userlib>:"Filter Error Codes__ogtk.vi"("Error In"=w395, "Error Codes to Filter"=w394) -> ("Error Out"=w396:errorcluster, "Filtered Error Details"=w393:T18)  [unwired: 7 in, 1 out]
        n200 = Unbundle(w393) -> ("code"=w391:i32, "source"=w392:string)
        n201 = Get Date/Time In Seconds() -> (seconds since 1Jan1904=w390:timestamp)
        n202 = Unbundle By Name(w386) -> ("Error Log"=w388:T2)
        n203 = Bundle By Name(cluster=T10 {"time"=timestamp(0 s since 1904-01-01), "code"=0, "source"=""} ("output cluster"), "time"=w390, "code"=w391, "source"=w392) -> (w387:T10)
        n204 = Build Array (concatenate)(w388, w387) -> (w384:T2)
        "Error List" <- w384
        n205 = Bundle By Name(cluster=w386, "Error Log"=w384) -> (w385:T12)
        n206 = call <vilib>:"General Error Handler.vi"("error in (no error)"=w396) -> ()  [unwired: 10 in, 5 out]
        n207 = call <vilib>:"Add State(s) to Queue__JKI_lib_State_Machine.vi"("State(s) in Front (\"\")"="/* Post Error States", "State(s) in (\"\")"=w400) -> ("States Out"=w399:string)  [unwired: 13 in]
      }
      frame "Exit" {
        # "Do not put any code in this frame.\n(No errors that occur here will be handled.)"
        n208 = call <vilib>:"Add State(s) to Queue__JKI_lib_State_Machine.vi"("State(s) in (\"\")"=w405) -> ("States Out"=w404:string)  [unwired: 14 in]
      }
      frame "---------- Data ----------" {
        # "Do not put any code in this frame.\n(It is a separator no-op. You can make a copy of this frame to create a new Data frame)"
        n209 = call <vilib>:"Add State(s) to Queue__JKI_lib_State_Machine.vi"("State(s) in (\"\")"=w409) -> ("States Out"=w408:string)  [unwired: 14 in]
      }
      frame "Data: Initialize" {
        w410 = refnum<visa-resource-name> "GPIB1::25::INSTR"  # IPS120 Address
        w411 = T2 []  # Error Log
        w413 = TRUE  # sentinel
        w414 = T19 {"Current VI Reference"=refnum, "Close Panel on Exit?"=FALSE}  # Core
        # "do not delete - used by framework"
        # "Data names and types of shift register data are defined by this bundle."
        # "Initialize the shift-register data, here.\n(data names are defined by what you wire into the bundle function)"
        n210 = Bundle("Core"=w414, "IPS120 Address"=w410, "sentinel"=w413, "Error Log"=w411) -> (w415:T12)  [unwired: 1 in]
        n211 = call <vilib>:"Add State(s) to Queue__JKI_lib_State_Machine.vi"("State(s) in (\"\")"=w417) -> ("States Out"=w416:string)  [unwired: 14 in]
      }
      frame "Data: Cleanup" {
        # "Cleanup any data and references, here.\n(this is called automatically, by the Macro: Exit)"
        n212 = Unbundle By Name(w418) -> ("Core.Current VI Reference"=w421:refnum<vi>)
        n213 = Close Reference(reference=w421, error in (no error)=w420) -> (error out=w419:errorcluster)
        n214 = call <vilib>:"Add State(s) to Queue__JKI_lib_State_Machine.vi"("State(s) in (\"\")"=w423) -> ("States Out"=w422:string)  [unwired: 14 in]
      }
      frame "---------- UI ----------" {
        # "Do not put any code in this frame.\n(It is a separator no-op. You can make a copy of this frame to create a new UI frame)"
        n215 = call <vilib>:"Add State(s) to Queue__JKI_lib_State_Machine.vi"("State(s) in (\"\")"=w427) -> ("States Out"=w426:string)  [unwired: 14 in]
      }
      frame "UI: Initialize" {
        w434 = FALSE
        # "start in local mode"
        # "Initialize the User Interface, here.\n(this is called automatically, by the Macro: Init)"
        n216 = disable-structure shown="Disabled" {
          frame Disabled {
            n217 = Open VI Reference(vi path=path "") -> ()  [unwired: 5 in, 2 out]
            n218 = call "MNK_Dashboard_v2.vi"() -> ()  [unwired: 12 in]
          }
          frame Enabled {
          }
        }
        n219 = Open Application Reference(8:w429) -> (0:w431:errorcluster, 3:w432:refnum<vi>)  [unwired: 3 in]
        n220 = property class="App"(reference=w432, error in=w431, "WebSrvr.Active"=TRUE ("Web Server:Server Active")) -> (error out=w428:errorcluster)  [unwired: 1 out]
        n221 = call <vilib>:"Add State(s) to Queue__JKI_lib_State_Machine.vi"("State(s) in (\"\")"=w439) -> ("States Out"=w438:string)  [unwired: 14 in]
        n222 = local write "Remote Mode"(w434) -> ()
        n223 = call "FGV - Attocube Remote.vi"("error in"=w428, "Function"=enum16{"write", "read"}."write", "Attocube Remote"=w434) -> ("error out"=w433:errorcluster)  [unwired: 3 in, 1 out]
        "Magnet Status 2" <- "" ("Magnet Status 2")
      }
      frame "UI: Cursor Set" {
        # "Argument"
        # "Set and Unset Cursor Busy.\n(Usage: \"UI: Cursor Set >> Busy|Idle\")"
        n224 = case shown="\"Idle\", Default" w441 {
          tunnel: w443 -> [w448 w450]
          tunnel: [w447 w449] -> w442
          frame "Idle", Default {
            n225 = call <vilib>:"Unset Busy.vi"("error in (no error)"=w448) -> ("error out"=w447:errorcluster)  [unwired: 10 in]
          }
          frame "Busy" {
            n226 = call <vilib>:"Set Busy.vi"("error in (no error)"=w450) -> ("error out"=w449:errorcluster)  [unwired: 9 in, 1 out]
          }
        }
        n227 = call <vilib>:"Add State(s) to Queue__JKI_lib_State_Machine.vi"("State(s) in (\"\")"=w446) -> ("States Out"=w445:string)  [unwired: 14 in]
      }
      frame "UI: Front Panel State" {
        # "Argument"
        # "Set Front Panel Open or Closed\n(Usage: \"UI: Front Panel State >> Open|Close\")"
        n228 = Unbundle By Name(w453) -> ("Core.Current VI Reference"=w452:refnum<vi>)
        n229 = case shown="\"Open\", Default" w451 {
          tunnel: w455 -> [w461 w474]
          tunnel: [w463 w475] -> w454
          tunnel: w452 -> [w462 w472]
          frame "Open", Default {
            n230 = property class="VI"(reference=w462, error in=w461) -> (reference out=w459:refnum<vi>, error out=w460:errorcluster, "Front Panel.Open"=w458:bool)
            n231 = case shown="True" w458 {
              tunnel: [w466 w469] -> w463
              tunnel: w460 -> [w465 w469]
              tunnel: w459 -> [w464 _]
              frame False {
                n232 = invoke class="VI" method="FP.Open"(reference=w464, error in=w465, "Activate"=TRUE, "State"=T11."Standard") -> (error out=w466:errorcluster)  [unwired: 1 in, 4 out]
              }
              frame True {
              }
            }
          }
          frame "Close" {
            n233 = property class="VI"(reference=w472, error in=w474) -> (reference out=w471:refnum<vi>, error out=w473:errorcluster, "Front Panel.Open"=w470:bool)
            n234 = case shown="True" w470 {
              tunnel: [w476 w479] -> w475
              tunnel: w473 -> [w476 w478]
              tunnel: w471 -> [_ w477]
              frame False {
              }
              frame True {
                n235 = invoke class="VI" method="FP.Close"(reference=w477, error in=w478) -> (error out=w479:errorcluster)  [unwired: 1 in, 2 out]
              }
            }
          }
        }
        n236 = call <vilib>:"Add State(s) to Queue__JKI_lib_State_Machine.vi"("State(s) in (\"\")"=w457) -> ("States Out"=w456:string)  [unwired: 14 in]
      }
      frame "---------- Macro ----------" {
        # "Do not put any code in this frame.\n(It is a separator no-op. You can make a copy of this frame to create a new Macro frame)"
        n237 = call <vilib>:"Add State(s) to Queue__JKI_lib_State_Machine.vi"("State(s) in (\"\")"=w483) -> ("States Out"=w482:string)  [unwired: 14 in]
      }
      frame "Macro: Initialize" {
        w484 = "Data: Initialize\nInitialize Core Data\nUI: Initialize\nUI: Front Panel State >> Open\nIPS120: Initialize"  # Data: Initialize Initialize Core Data UI: Initialize UI: Front Panel State >> Open IPS120: Initialize
        # "Initialization Macro\n(This is called once, when the VI starts)"
        n238 = call <vilib>:"Add State(s) to Queue__JKI_lib_State_Machine.vi"("State(s) in Front (\"\")"=w484, "State(s) in (\"\")"=w488) -> ("States Out"=w487:string)  [unwired: 13 in]
      }
      frame "Macro: Exit" {
        # "Exit Macro\n(This is called once, when the VI exits)"
        n239 = Unbundle By Name(w501) -> ("Core.Close Panel on Exit?"=w500:bool, "Mercury ITC Ref"=w493, "Mercury IPS Ref"=w492)
        n240 = call <instrlib>:"Close.vi"("error in (no error)"=w491, "Mercury Reference"=w492) -> ("error out"=w490:errorcluster)  [unwired: 9 out]
        n241 = call <instrlib>:"Close.vi"("error in (no error)"=w490, "Mercury Reference"=w493) -> ("error out"=w494:errorcluster)  [unwired: 9 out]
        n242 = call <vilib>:"Simple Error Handler.vi"("error in (no error)"=w494) -> ("error out"=w489:errorcluster)  [unwired: 1 in, 7 out]
        n243 = Select(t="UI: Front Panel State >> Close", s=w500, f="") -> (s? t:f=w497:string)
        n244 = call <vilib>:"Add State(s) to Queue__JKI_lib_State_Machine.vi"("State(s) in (\"\")"=w497, "State(s) at Back (\"\")"="Data: Cleanup\nExit") -> ("States Out"=w495:string)  [unwired: 13 in]
        n245 = call <vilib>:"Add State(s) to Queue__JKI_lib_State_Machine.vi"("State(s) in Front (\"\")"=w495, "State(s) in (\"\")"=w503) -> ("States Out"=w502:string)  [unwired: 13 in]
      }
      frame "---------- New Category ----------" {
        n246 = call <vilib>:"Add State(s) to Queue__JKI_lib_State_Machine.vi"("State(s) in (\"\")"=w507) -> ("States Out"=w506:string)  [unwired: 14 in]
      }
      frame "IPS120: Initialize" {
        n247 = call "NI USB GPIB Command.vi"("Error In"=w511, "String to Send"="C3", "VISA resource name"="IPS120 Address") -> ("Error Out"=w510:errorcluster)  [unwired: 1 in, 3 out]
        n248 = Bundle By Name(cluster=w514, "IPS120 Address"="IPS120 Address") -> (w513:T12)
        n249 = call <vilib>:"Add State(s) to Queue__JKI_lib_State_Machine.vi"("State(s) in (\"\")"=w516, "State(s) at Back (\"\")"="Mercury: Query ITC: System\nMercury: Query IPS: System\nMercury: Query ITC: Temperature\nMercury: Query ITC: Heater\nMercury: Query ITC: Aux\nMercury: Query ITC: Pressure\nMercury: Query IPS: LVL\nMercury: Query IPS: Temperature\nMercury: Query IPS: Magnet" ("State(s) at Back (\"\")")) -> ("States Out"=w515:string)  [unwired: 13 in]
      }
      frame "IPS120: Idle" {
        n250 = Unbundle By Name(w550) -> ("IPS120 Address"=w524:refnum<visa-resource-name>)
        n251 = call "IPS Read Magnet Field.vi"("Error In"=w523, "VISA resource name"=w524) -> ("Error Out"=w542:errorcluster, "Magnet FIeld (T)"=w543:dbl, "VISA resource name"=w541:refnum<visa-resource-name>)  [unwired: 1 in]
        "Magnet Field (T)" <- w543
        "Magnet Field (T)" <- w543
        n252 = call "IPS Read Set Point Field.vi"("Error In"=w542, "VISA resource name"=w541) -> ("Error Out"=w539:errorcluster, "Set Point (T)"=w540:dbl, "VISA resource name"=w538:refnum<visa-resource-name>)  [unwired: 1 in]
        "Target Field (T)" <- w540
        n253 = call "IPS Examine Status.vi"("Error In"=w523, "VISA resource name 2"=w524) -> ("Return String from Device (Not all commands return a String)"=w522:string)  [unwired: 1 in, 2 out]
        n254 = call "IPS Read PS Current.vi"("Error In"=w539, "VISA resource name"=w538) -> ("Error Out"=w537:errorcluster, "Current (A)"=w526:dbl, "VISA resource name"=w536:refnum<visa-resource-name>)  [unwired: 1 in]
        "Current (A)" <- w526
        "Current (A)" <- w526
        n255 = call "IPS Read PS Field.vi"("Error In"=w537, "VISA resource name (COM Port of Prologix Device)"=w536) -> ("Error Out"=w534:errorcluster, "Field (T)"=w535:dbl, "VISA resource name (COM Port of Prologix Device) 2"=w533:refnum<visa-resource-name>)  [unwired: 1 in]
        "Power Supply Field (T)" <- w535
        n256 = call "IPS Get Status.vi"("Return String from Device (Not all commands return a String)"=w522) -> ("System"=w519:string, "SHeater"=w520:string, "Mode"=w521:string, "Activity"=w518:string)  [unwired: 7 in]
        "Magnet Status" <- w518
        n257 = call "IPS Read PS Voltage.vi"("Error In"=w534, "VISA resource name"=w533) -> ("Error Out"=w531:errorcluster, "Power Supplly Voltage"=→"Voltage (V)" →"Voltage (V)":dbl, "VISA resource name"=w529:refnum<visa-resource-name>)  [unwired: 1 in]
        n258 = call "IPS Read Field Sweep Rate.vi"("Error In"=w531, "VISA resource name"=w529) -> ("Field Sweep Rate (T/min)"=w530:dbl)  [unwired: 1 in, 2 out]
        "Target Field Rate (T/min)" <- w530
        n259 = Build Array(w543, w540, w526, w535, w530) -> (w528:dbl[])
        n260 = call "FGV_PSP - IPS120 Status.vi"("Function"=enum16{"write", "read"}."read") -> ("error out"=w547:errorcluster, "status"=w545:T20)  [unwired: 5 in]
        n261 = Bundle By Name(cluster=w545) -> (w544:T20)  [unwired: 1 in]
        n262 = Build Array(w518, w521, w520, w519) -> (w527:string[])
        n263 = call "FGV_PSP - IPS120 Status.vi"("error in"=w547, "Function"=enum16{"write", "read"}."write", "status"=w544) -> ("error out"=w546:errorcluster)  [unwired: 3 in, 1 out]
        n264 = call "IPS120_to_DSC.vi"("str"=w527, "str var"=refnum<k21>[] ["ni.var.psp://housesoftheholy/DR200/DR200_Magnet_Status_Activity", "ni.var.psp://housesoftheholy/DR200/DR200_Magnet_Status_Mode", "ni.var.psp://housesoftheholy/DR200/DR200_Magnet_Status_Switch_Heater", "ni.var.psp://housesoftheholy/DR200/DR200_Magnet_Status_System"], "dbl"=w528, "dbl var"=refnum<k21>[] ["ni.var.psp://housesoftheholy/DR200/DR200_Magnet_Field", "ni.var.psp://housesoftheholy/DR200/DR200_Magnet_Field_Target", "ni.var.psp://housesoftheholy/DR200/DR200_Magnet_PS_Current", "ni.var.psp://housesoftheholy/DR200/DR200_Magnet_PS_Field", "ni.var.psp://housesoftheholy/DR200/DR200_Magnet_PS_Voltage", "ni.var.psp://housesoftheholy/DR200/DR200_Magnet_Rate_Target"]) -> ()
        n265 = call <vilib>:"Add State(s) to Queue__JKI_lib_State_Machine.vi"("State(s) in (\"\")"=w551) -> ("States Out"=w552:string)  [unwired: 14 in]
      }
      frame "IPS120: Empty" {
        n266 = Unbundle By Name(w554) -> ()  [unwired: 1 out]
        n267 = call <vilib>:"Add State(s) to Queue__JKI_lib_State_Machine.vi"("State(s) in (\"\")"=w555) -> ("States Out"=w556:string)  [unwired: 14 in]
      }
    }
  }
  n268 = disable-structure shown="Disabled" {
    frame Disabled {
      (unwired) FALSE
      n269 = disable-structure shown="Disabled" {
        frame Disabled {
          n270 = property on="Fast/Slow Fill" class="Bool (strict)" props=["Val(Sgnl)"]() -> ()  [unwired: 3 in, 2 out]
        }
        frame Enabled {
        }
      }
      n271 = local read "PS Heat"() -> ()  [unwired: 1 in]
      n272 = local read "Lambda"() -> ()  [unwired: 1 in]
    }
    frame Enabled {
    }
  }
